vi "Create HDF File.vi"(7 "Dims":u64[](array[numeric]), 8 "error in (no error)":errorcluster, 10 "variant":variant, 11 "path":string) -> (0 "error out":errorcluster, 3 "path out":path)   [LabVIEW 2019, in "HDF5 Tools.lvlib"]
uses:
  HDF5 Tools.lvlib
  <vilib>/UPVI/lvhdf5/file.llb/LVH5F Operation.ctl
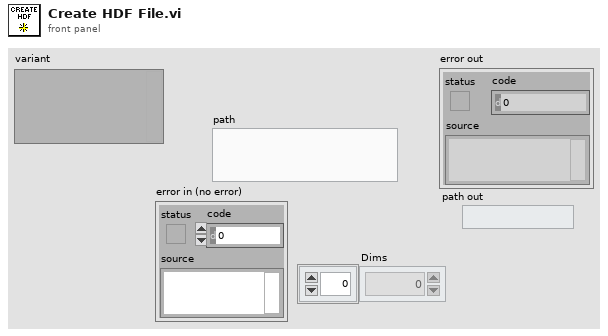
[diagram p1: front panel]
types:
  T1 = typedef "LVH5F Operation.ctl" = enum16{"open", "open or create", "create or replace", "create or replace (with confirmation)", "create", "open (read only)"}
  T2 = typedef "HDF5 Ref.ctl" = refnum<k1>
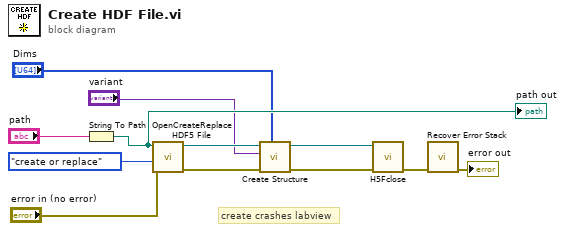
[diagram p0: block diagram]
diagram:
  # "create crashes labview"
  n1 = String To Path(string="path") -> (path=w3:path)
  "path out" <- w3
  n2 = call <vilib>:"OpenCreateReplace HDF5 File.vi"("error in (no error)"="error in (no error)", "function (open or create)"=LVH5F_Operation."create or replace", "path"=w3) -> ("error out"=w8:errorcluster, "HDF5 Ref out"=w9:T2)  [unwired: 5 in]
  n3 = call "Create Structure.vi"("Dims"="Dims", "error in (no error)"=w8, "variant"="variant", "Refnum in"=w9) -> ("error out"=w7:errorcluster, "Refnum out"=w4:T2)  [unwired: 4 in]
  n4 = call <vilib>:"H5Fclose.vi"("error in (no error)"=w7, "HDF5 Ref"=w4) -> ("error out"=w12:errorcluster)  [unwired: 7 in]
  n5 = call <vilib>:"Recover Error Stack.vi"("error in (no error)"=w12) -> ("error out"=→"error out":errorcluster)  [unwired: 5 in, 3 out]
